vi "(SubVI)_2Dstart_BD_ver9_two_daqs.vi"(0 "Master Ctr (Ctr0)":tag, 1 "Master Ctr Terminal (PFI0)":tag, 2 "Galvo Hardware":T2, 3 "Camera Hardware":T1, 4 "input cluster":T3, 5 "error in (no error)":errorcluster, 6 "B-Scan Frequency":dbl=100.0, 7 "A-scans per Image":u32, 8 "Camera Delay (us)":dbl format="%.6f") -> (13 "Image Size":u32, 14 "Master Ctr Task Out":refnum<k21>, 15 "Galvo AO Task Out":refnum<k21>, 16 "Camera Ctr Task Out":refnum<k21>, 17 "Galvo Ctr Task Out":refnum<k21>, 18 "output cluster":T3, 19 "AO Err Out":errorcluster)   [LabVIEW 2019]
uses:
  <vilib>/DAQmx/write.llb/DAQmx Write (Analog 2D DBL NChan NSamp).vi
  <vilib>/DAQmx/create/channels.llb/DAQmx Create Channel (CO-Pulse Generation-Frequency).vi
  <vilib>/DAQmx/configure/timing.llb/DAQmx Timing (Implicit).vi
  <vilib>/DAQmx/configure/trigger.llb/DAQmx Start Trigger (Digital Edge).vi
  <vilib>/DAQmx/create/channels.llb/DAQmx Create Channel (AO-Voltage-Basic).vi
  <vilib>/DAQmx/configure/timing.llb/DAQmx Timing (Sample Clock).vi
  <vilib>/DAQmx/miscellaneous.llb/DAQmx Fill In Error Info.vi
  <resource>/objmgr/daqmx.rc
panel:
  out "B-Scan Frequency 2":dbl
  in  "counter":tag
  out "error out":errorcluster
  out "task out":refnum<k21>
  in  "2D frequency":i16
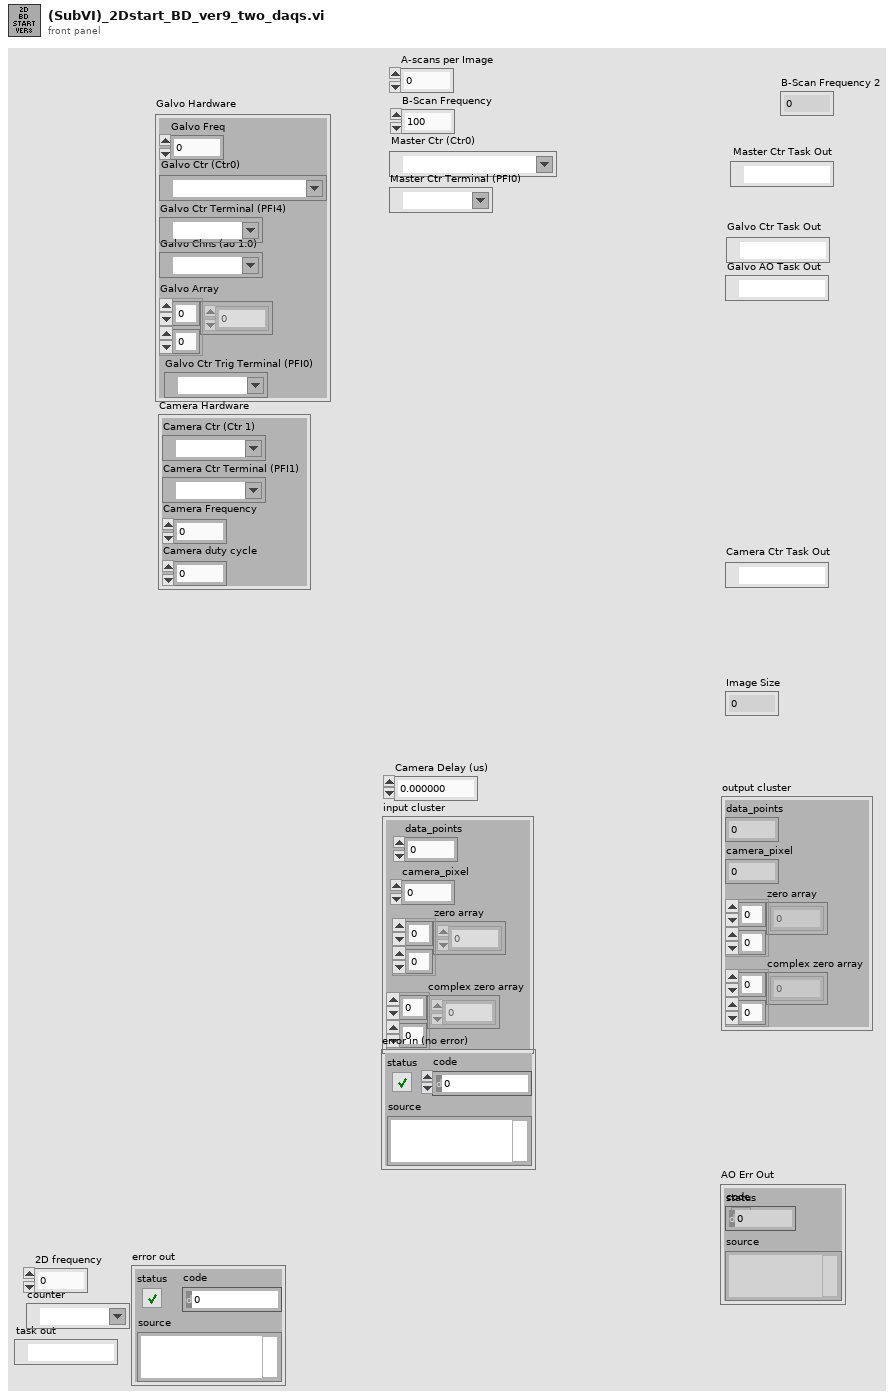
[diagram p1: front panel]
types:
  T1 = cluster{"Camera Ctr (Ctr 1)":tag, "Camera Ctr Terminal (PFI1)":tag, "Camera Frequency":dbl, "Camera duty cycle":dbl}
  T2 = cluster{"Galvo Array":dbl[][], "Galvo Chns (ao 1:0)":tag, "Galvo Ctr (Ctr0)":tag, "Galvo Ctr Terminal (PFI4)":tag, "Galvo Freq":dbl, "Galvo Ctr Trig Terminal (PFI0)":tag}
  T3 = cluster{"data_points":i32, "camera_pixel":i32, "zero array":dbl[][], "complex zero array":dbl[][]}
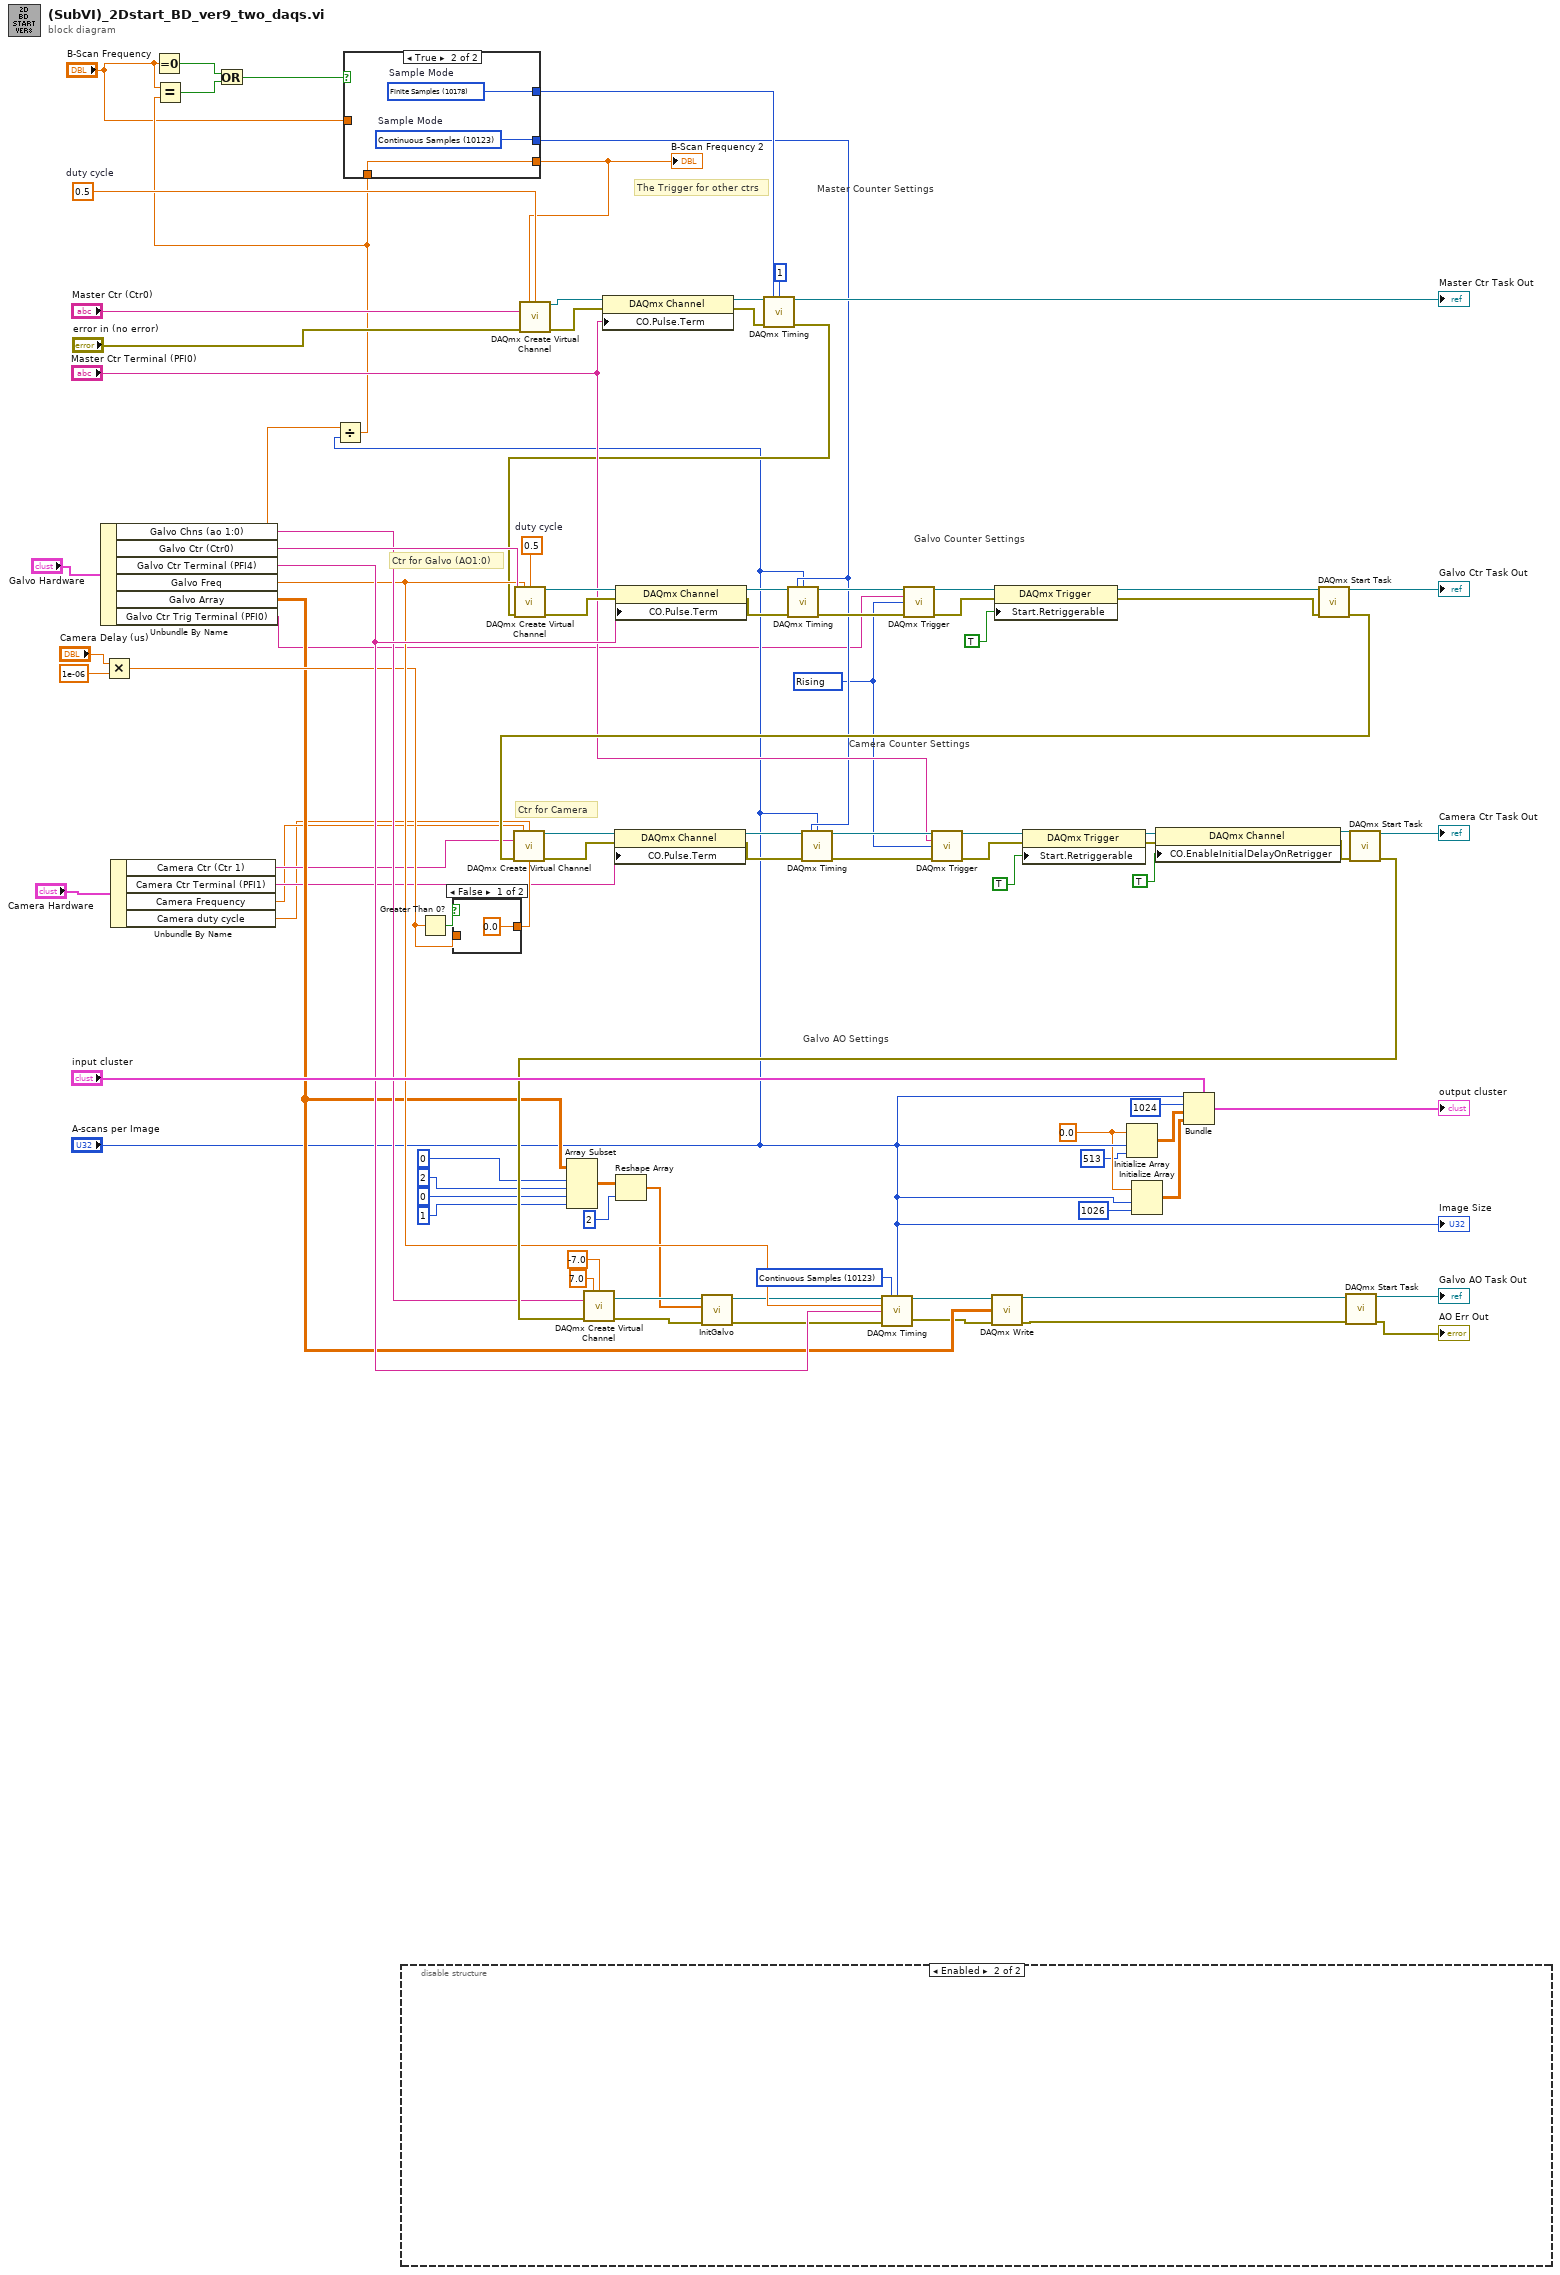
[diagram p0: block diagram]
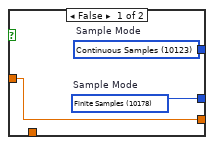
[diagram p3: hidden frame]
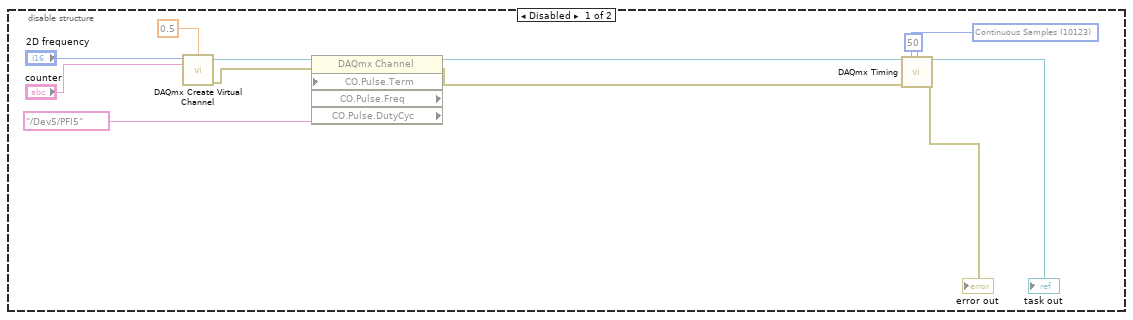
[diagram p4: hidden frame]
diagram:
  w25 = 0.0 ("element")
  w20 = 10123 items=["Finite Samples"=10178, "Continuous Samples"=10123, "Hardware Timed Single Point"=12522] ("sample mode")
  w44 = 10280 items=["Rising"=10280, "Falling"=10171] ("edge")
  w87 = 0.5  # duty cycle
  w92 = 0.5  # duty cycle
  # "Galvo AO Settings"
  # "Camera Counter Settings"
  # "Galvo Counter Settings"
  # "Master Counter Settings"
  # "Ctr for Camera"
  # "Ctr for Galvo (AO1:0)"
  # "The Trigger for other ctrs"
  n1 = Unbundle By Name("Galvo Hardware") -> ("Galvo Chns (ao 1:0)"=w64:tag, "Galvo Ctr (Ctr0)"=w66:tag, "Galvo Ctr Terminal (PFI4)"=w67:tag, "Galvo Freq"=w56:dbl, "Galvo Array"=w43:dbl[][], "Galvo Ctr Trig Terminal (PFI0)"=w5:tag)
  n2 = Multiply(x="Camera Delay (us)", y=1e-06) -> (x*y=w51:dbl)
  n3 = Unbundle By Name("Camera Hardware") -> ("Camera Ctr (Ctr 1)"=w41:tag, "Camera Ctr Terminal (PFI1)"=w40:tag, "Camera Frequency"=w39:dbl, "Camera duty cycle"=w38:dbl)
  n4 = Equal To 0?(x="B-Scan Frequency") -> (x = 0?=w35:bool)
  n5 = Divide(x=w56, y="A-scans per Image") -> (x/y=w37:dbl)
  n6 = Equal?(x="B-Scan Frequency", y=w37) -> (x = y?=w34:bool)
  n7 = Or(x=w35, y=w34) -> (x .or. y?=w33:bool)
  n8 = case shown="True" w33 {
    tunnel: "B-Scan Frequency" -> [w99 _]
    tunnel: [w99 w102] -> w48
    tunnel: w37 -> [_ w102]
    tunnel: [w98 w101] -> w47
    tunnel: [w97 w100] -> w45
    frame False {
      w97 = 10178 items=["Finite Samples"=10178, "Continuous Samples"=10123, "Hardware Timed Single Point"=12522]  # Sample Mode
      w98 = 10123 items=["Finite Samples"=10178, "Continuous Samples"=10123, "Hardware Timed Single Point"=12522]  # Sample Mode
    }
    frame True {
      w100 = 10123 items=["Finite Samples"=10178, "Continuous Samples"=10123, "Hardware Timed Single Point"=12522]  # Sample Mode
      w101 = 10178 items=["Finite Samples"=10178, "Continuous Samples"=10123, "Hardware Timed Single Point"=12522]  # Sample Mode
    }
  }
  "B-Scan Frequency 2" <- w48
  n9 = disable-structure shown="Enabled" {
    frame Disabled {
      w111 = 10123 items=["Finite Samples"=10178, "Continuous Samples"=10123, "Hardware Timed Single Point"=12522] ("sample mode")
      n10 = call-poly <vilib>:"DAQmx Create Virtual Channel.vi"("frequency"="2D frequency", "duty cycle"=0.5, "counter"="counter") -> ("task out"=w107:refnum<k21>, "error out"=w106:errorcluster)  [unwired: 6 in, 5 out]
      n11 = property class="DAQmx Channel" props=["CO.Pulse.Term", "CO.Pulse.Freq", "CO.Pulse.DutyCyc"](reference=w107, error in=w106, "CO.Pulse.Term"=tag "/Dev5/PFI5") -> (reference out=w105:refnum<k21>, error out=w104:errorcluster)  [unwired: 2 out]
      n12 = call-poly <vilib>:"DAQmx Timing.vi"("task/channels in"=w105, "sample mode"=w111, "samples per channel"=50, "error in"=w104) -> ("task out"=→"task out":refnum<k21>, "error out"=→"error out":errorcluster)  [unwired: 2 in, 8 out]
    }
    frame Enabled {
    }
  }
  n13 = Greater Than 0?(x=w51) -> (x > 0?=w55:bool)
  n14 = case shown="False" w55 {
    tunnel: w51 -> [_ w116]
    tunnel: [0.0 ("Camera Delay") w116] -> w54
    frame False {
    }
    frame True {
    }
  }
  n15 = call-poly <vilib>:"DAQmx Create Virtual Channel.vi"("frequency"=w48, "duty cycle"=w92, "counter"="Master Ctr (Ctr0)", "error in"="error in (no error)") -> ("task out"=w95:refnum<k21>, "error out"=w94:errorcluster)  [unwired: 10 in]
  n16 = Array Subset(array=w43, index (row)=0 ("index"), length (row)=2 ("length"), index (col)=0 ("index"), length (col)=1 ("length")) -> (w15:dbl[][])
  n17 = property class="DAQmx Channel"(reference=w95, error in=w94, "CO.Pulse.Term"="Master Ctr Terminal (PFI0)") -> (reference out=w91:refnum<k21>, error out=w90:errorcluster)
  n18 = Reshape Array(w15, 2 ("dimension size")) -> (w10:dbl[])
  n19 = call-poly <vilib>:"DAQmx Timing.vi"("task/channels in"=w91, "sample mode"=w47, "samples per channel"=1, "error in"=w90) -> ("task out"=→"Master Ctr Task Out":refnum<k21>, "error out"=w50:errorcluster)  [unwired: 10 in]
  n20 = call-poly <vilib>:"DAQmx Create Virtual Channel.vi"("frequency"=w56, "duty cycle"=w87, "counter"=w66, "error in"=w50) -> ("task out"=w89:refnum<k21>, "error out"=w88:errorcluster)  [unwired: 10 in]
  n21 = property class="DAQmx Channel"(reference=w89, error in=w88, "CO.Pulse.Term"=w67) -> (reference out=w76:refnum<k21>, error out=w75:errorcluster)
  n22 = call-poly <vilib>:"DAQmx Timing.vi"("task/channels in"=w76, "sample mode"=w45, "samples per channel"="A-scans per Image", "error in"=w75) -> ("task out"=w74:refnum<k21>, "error out"=w73:errorcluster)  [unwired: 10 in]
  n23 = call-poly <vilib>:"DAQmx Trigger.vi"("task/channels in"=w74, "source"=w5, "edge"=w44, "error in"=w73) -> ("task out"=w85:refnum<k21>, "error out"=w86:errorcluster)  [unwired: 10 in]
  n24 = property class="DAQmx Trigger"(reference=w85, error in=w86, "Start.Retriggerable"=TRUE) -> (reference out=w4:refnum<k21>, error out=w3:errorcluster)
  n25 = Initialize Array(w25, "A-scans per Image", 513 ("dimension size")) -> (w23:dbl[][])
  n26 = Initialize Array(w25, "A-scans per Image", 1026 ("dimension size")) -> (w24:dbl[][])
  n27 = Bundle(cluster="input cluster", "data_points"="A-scans per Image", "camera_pixel"=1024, "zero array"=w23, "complex zero array"=w24) -> (→"output cluster":T3)
  n28 = call <vilib>:"DAQmx Start Task.vi"("task/channels in"=w4, "error in"=w3) -> ("task out"=→"Galvo Ctr Task Out":refnum<k21>, "error out"=w68:errorcluster)  [unwired: 12 in]
  n29 = call-poly <vilib>:"DAQmx Create Virtual Channel.vi"("frequency"=w39, "duty cycle"=w38, "counter"=w41, "error in"=w68, "initial delay"=w54) -> ("task out"=w82:refnum<k21>, "error out"=w81:errorcluster)  [unwired: 9 in]
  n30 = property class="DAQmx Channel"(reference=w82, error in=w81, "CO.Pulse.Term"=w40) -> (reference out=w72:refnum<k21>, error out=w71:errorcluster)
  n31 = call-poly <vilib>:"DAQmx Timing.vi"("task/channels in"=w72, "sample mode"=w45, "samples per channel"="A-scans per Image", "error in"=w71) -> ("task out"=w70:refnum<k21>, "error out"=w69:errorcluster)  [unwired: 10 in]
  n32 = call-poly <vilib>:"DAQmx Trigger.vi"("task/channels in"=w70, "source"="Master Ctr Terminal (PFI0)", "edge"=w44, "error in"=w69) -> ("task out"=w79:refnum<k21>, "error out"=w80:errorcluster)  [unwired: 10 in]
  n33 = property class="DAQmx Trigger"(reference=w79, error in=w80, "Start.Retriggerable"=TRUE) -> (reference out=w62:refnum<k21>, error out=w61:errorcluster)
  n34 = property class="DAQmx Channel"(reference=w62, error in=w61, "CO.EnableInitialDelayOnRetrigger"=TRUE) -> (reference out=w59:refnum<k21>, error out=w58:errorcluster)
  n35 = call <vilib>:"DAQmx Start Task.vi"("task/channels in"=w59, "error in"=w58) -> ("task out"=→"Camera Ctr Task Out":refnum<k21>, "error out"=w65:errorcluster)  [unwired: 12 in]
  n36 = call-poly <vilib>:"DAQmx Create Virtual Channel.vi"("maximum value"=7.0, "minimum value"=-7.0, "physical channels"=w64, "error in"=w65) -> ("task out"=w11:refnum<k21>, "error out"=w14:errorcluster)  [unwired: 5 in, 5 out]
  n37 = call "InitGalvo.vi"("error in"=w14, "Output Array"=w10, "task/channels in"=w11) -> ("error out"=w13:errorcluster, "task out"=w12:refnum<k21>)  [unwired: 7 in]
  n38 = call-poly <vilib>:"DAQmx Timing.vi"("task/channels in"=w12, "sample mode"=w20, "samples per channel"="A-scans per Image", "rate"=w56, "source"=w67, "error in"=w13) -> ("task out"=w19:refnum<k21>, "error out"=w27:errorcluster)  [unwired: 1 in, 7 out]
  n39 = call-poly <vilib>:"DAQmx Write.vi"("task/channels in"=w19, "data"=w43, "error in"=w27) -> ("task out"=w2:refnum<k21>, "error out"=w1:errorcluster)  [unwired: 1 in, 10 out]
  n40 = call <vilib>:"DAQmx Start Task.vi"("task/channels in"=w2, "error in"=w1) -> ("task out"=→"Galvo AO Task Out":refnum<k21>, "error out"=→"AO Err Out":errorcluster)  [unwired: 12 in]
  "Image Size" <- "A-scans per Image"
